vi "niDTS GNSS RF Test Set Parameters.vi"(0 "Template Tx Test Handle in":T2, 7 "Parameters":T1 {"External Attenuation (dB)" format="%.1g"; "Power (dBm)" format="%.1g"}, 11 "error in (no error)":errorcluster) -> (4 "Template Tx Test Handle out":T2, 15 "error out":errorcluster)   [LabVIEW 2014, in "niDTS GNSS.lvlib"]
uses:
  niDTS GNSS.lvlib
  Includes/niDTS GNSS RF Test INC Handle.ctl
  Objects/BASE_class/niDTS GNSS RF Test.lvclass
  Includes/niDTS GNSS RF Test INC Parameters.ctl
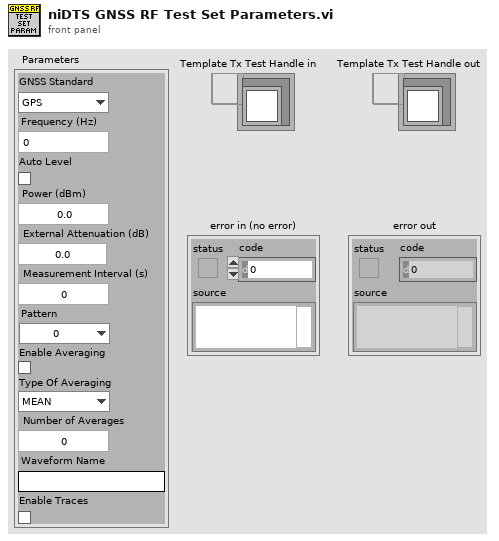
[diagram p1: front panel]
types:
  T1 = typedef "niDTS GNSS.lvlib/niDTS GNSS RF Test INC Parameters.ctl" = cluster{"GNSS Standard":enum16{"GPS", "GLONASS", "Galileo", "Beidou"}, "Frequency (Hz)":dbl, "Auto Level":bool, "Power (dBm)":dbl, "External Attenuation (dB)":dbl, "Measurement Interval (s)":dbl, "Pattern":enum16{"0", "1", "01", "00001111", "PN9"}, "Enable Averaging":bool, "Type Of Averaging":enum16{"MEAN", "MAX", "MIN", "MAXMIN"}, "Number of Averages":i32, "Waveform Name":string, "Enable Traces":bool}
  T2 = typedef "niDTS GNSS.lvlib/niDTS GNSS RF Test INC Handle.ctl" = refnum<data-value>
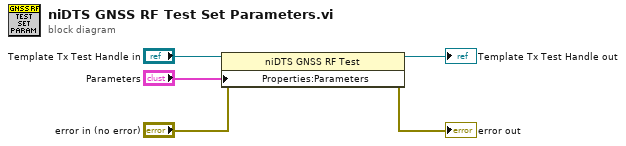
[diagram p0: block diagram]
diagram:
  n1 = property class="niDTS GNSS RF Test"(reference="Template Tx Test Handle in", error in="error in (no error)", "Properties:Parameters"="Parameters") -> (reference out=→"Template Tx Test Handle out":T2, error out=→"error out":errorcluster)
